vi "Get.vi"(8 "error in (no error)":errorcluster, 11 "Instrument in":refnum<class "Instrument.lvclass">) -> (0 "error out":errorcluster, 2 "Numeric":dbl, 3 "Instrument out":refnum<class "Instrument.lvclass">)   [LabVIEW 2018, in "Instrument.lvclass"]
uses:
  Instrument.lvclass
  Instrument.lvclass/Instrument.ctl
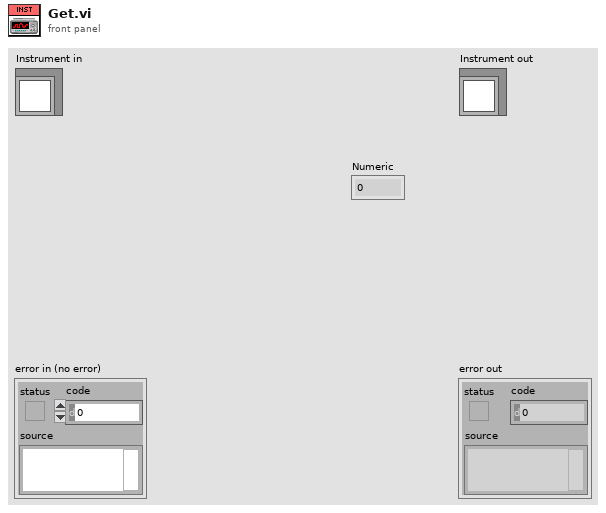
[diagram p1: front panel]
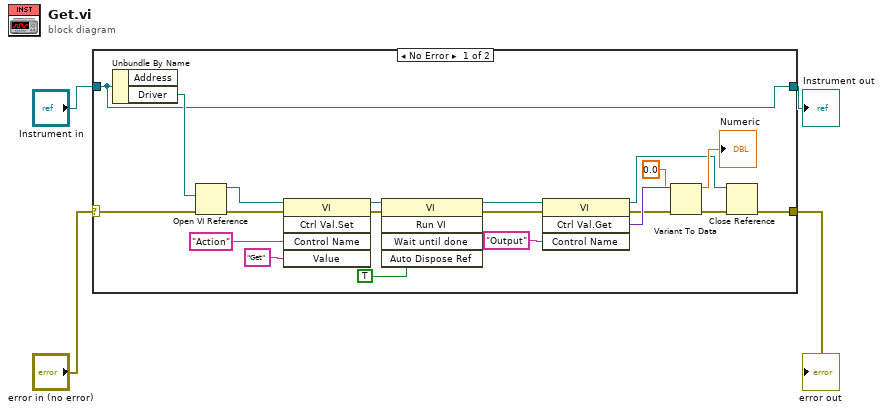
[diagram p0: block diagram]
diagram:
  n1 = case shown="No Error" "error in (no error)" {
    selector: "error in (no error)" -> [w18 w26]
    tunnel: [w6 w26] -> w3
    tunnel: [w19 w25] -> w1
    tunnel: "Instrument in" -> [w19 w25]
    frame No Error {
      n2 = Unbundle By Name(w19) -> ("Driver"=w24:path)  [unwired: 1 out]
      n3 = Open VI Reference(vi path=w24, error in (no error)=w18) -> (vi reference=w20:refnum<vi>, error out=w21:errorcluster)  [unwired: 4 in]
      n4 = invoke class="VI" method="Ctrl Val.Set"(reference=w20, error in=w21, "Control Name"="Action", "Value"="Get" ("Control Name")) -> (reference out=w17:refnum<vi>, error out=w16:errorcluster)  [unwired: 1 in, 3 out]
      n5 = invoke class="VI" method="Run VI"(reference=w17, error in=w16, "Wait until done"=TRUE ("Wait Until Done")) -> (reference out=w14:refnum<vi>, error out=w13:errorcluster)  [unwired: 2 in, 3 out]
      n6 = invoke class="VI" method="Ctrl Val.Get"(reference=w14, error in=w13, "Control Name"="Output") -> (reference out=w8:refnum<vi>, error out=w9:errorcluster, "Get Control Value Variant"=w12:variant)  [unwired: 1 in, 1 out]
      n7 = Variant To Data(error in=w9, type=0.0 ("Numeric 2"), Variant=w12) -> (data=→"Numeric":dbl, error out=w7:errorcluster)
      n8 = Close Reference(reference=w8, error in (no error)=w7) -> (error out=w6:errorcluster)
    }
    frame Error {
    }
  }
  "error out" <- w3
  "Instrument out" <- w1
